vi "laser.vi"(8 "error in (no error)":errorcluster, 11 "this module name":string) -> (0 "error out":errorcluster)   [LabVIEW 2019]
doc: "Communicates with a laser to set the output power."
uses:
  common/common data types/common_event_data.ctl
panel:
  out "global stop?":bool
  in  "stop this module":bool
  out "targetted":bool
  out "msg target":string
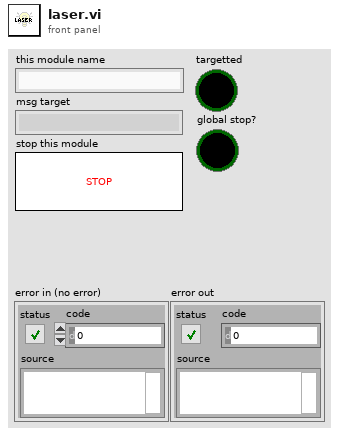
[diagram p1: front panel]
types:
  T1 = typedef "common_event_data.ctl" = cluster{"sender":string, "target":string, "msg":string, "data":variant}
  T2 = cluster{"this module name":string, "laser SP":dbl}
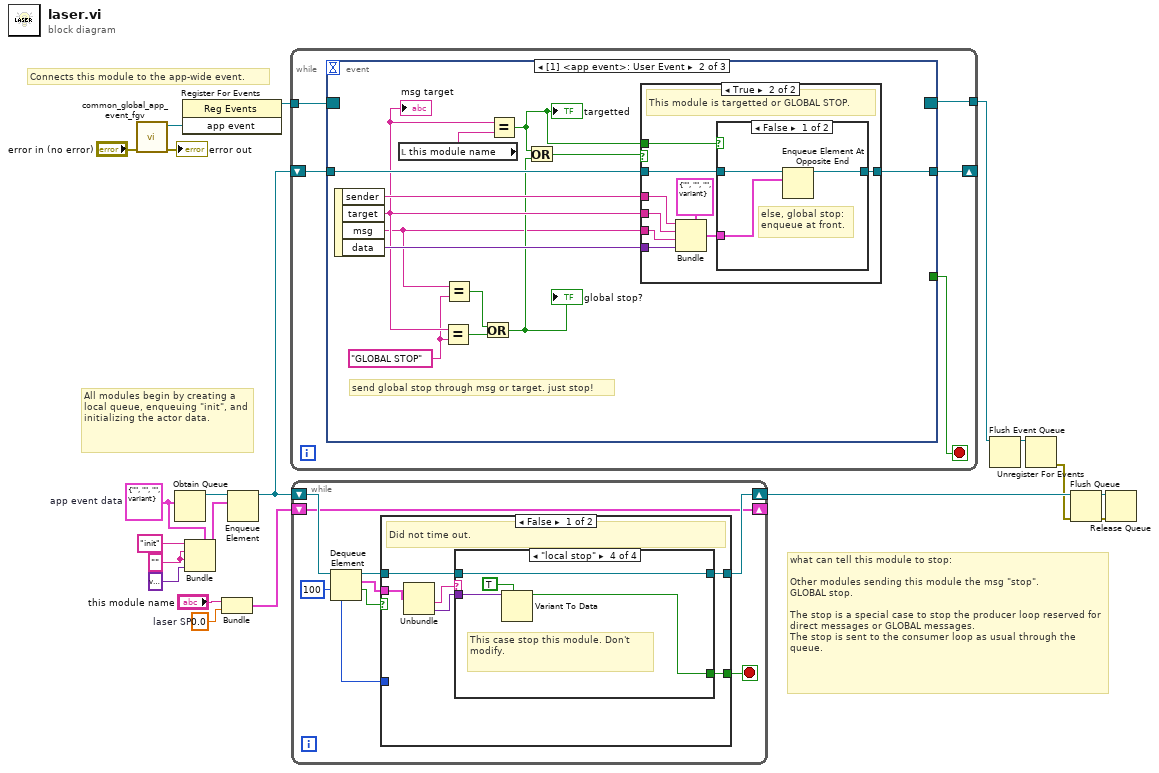
[diagram p0: block diagram]
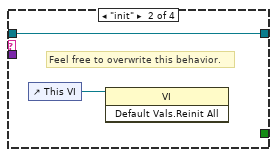
[diagram p3: hidden frame]
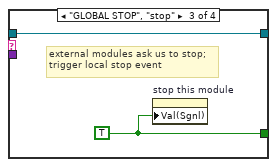
[diagram p4: hidden frame]
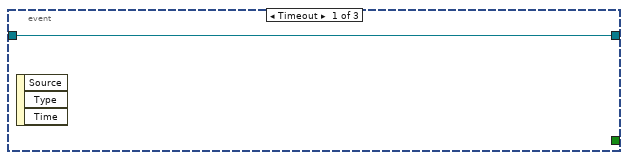
[diagram p6: hidden frame]
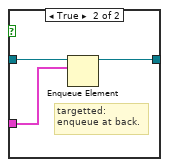
[diagram p8: hidden frame]
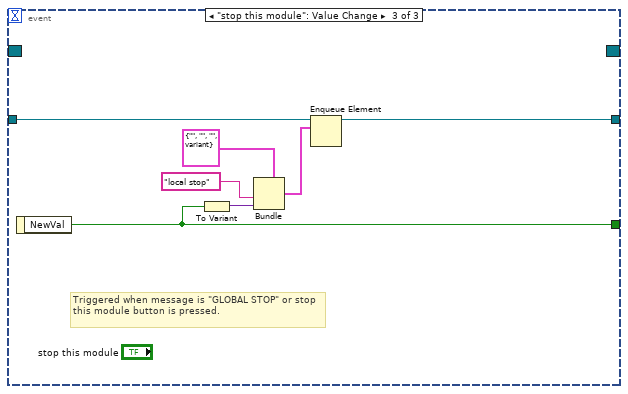
[diagram p9: hidden frame]
diagram:
  w1 = 0.0  # laser SP
  w6 = "" ("target")
  w8 = T1 {"sender"="", "target"="", "msg"="", "data"=variant}  # app event data
  # "All modules begin by creating a local queue, enqueuing \"init\", and initializing the actor data."
  # "what can tell this module to stop:\n\nOther modules sending this module the msg \"stop\".\nGLOBAL stop.\n\nThe stop is a special case to stop the producer loop reserved for direct messages or GLOBAL messages.\nThe stop is sent to the consumer loop as usual through the queue."
  # "Connects this module to the app-wide event."
  n1 = call "common_global_app_event_fgv.vi"("error in (no error)"="error in (no error)") -> ("error out"=→"error out":errorcluster, "app event"=w13:refnum<user-event>)  [unwired: 9 in]
  n2 = Obtain Queue(element data type=w8) -> (queue out=w20:refnum<queue>)  [unwired: 4 in, 2 out]
  n3 = register-events(w13) -> (reference out=w14:refnum<event-registration>)  [unwired: 2 in, 1 out]
  n4 = Bundle(cluster=w8, "sender"="init" ("msg"), "target"=w6, "msg"=w6, "data"=variant) -> (w18:T1)
  n5 = Bundle("this module name"="this module name", "laser SP"=w1) -> (w4:T2)  [unwired: 1 in]
  n6 = Enqueue Element(queue=w20, element=w18) -> (queue out=w17:refnum<queue>)  [unwired: 2 in, 2 out]
  n7 = while {
    tunnel: w14 -> [w25]
    shift-right: [w23] -> _
    shift-left: w17 -> [w24]
    tunnel: [w22] -> w3
    stop <- w21 stop-if-true
    n8 = event shown="[1] <app event>: User Event" {
      selector: w25 -> [_ _ _]
      dyn-events: [_ _ _] -> w22
      timeout: _ -> [_ _ _]
      tunnel: w24 -> [w26 w38 w60]
      tunnel: [w26 w37 w61] -> w23
      tunnel: [_ _ w56] -> w21
      event Timeout {
        n9 = event-data() -> ()  [unwired: 1 in, 3 out]
      }
      event User Event {
        w30 = "GLOBAL STOP"
        # "send global stop through msg or target. just stop!"
        n10 = event-data() -> ("sender"=w36:string, "target"=w35:string, "msg"=w29:string, "data"=w39:variant)  [unwired: 1 in]
        "msg target" <- w35
        n11 = local read "this module name"() -> (w27:string)
        n12 = Equal?(x=w35, y=w30) -> (x = y?=w32:bool)
        n13 = Equal?(x=w29, y=w30) -> (x = y?=w28:bool)
        n14 = Or(x=w28, y=w32) -> (x .or. y?=w31:bool)
        "global stop?" <- w31
        n15 = Equal?(x=w35, y=w27) -> (x = y?=w33:bool)
        "targetted" <- w33
        n16 = Or(x=w33, y=w31) -> (x .or. y?=w34:bool)
        n17 = case shown="True" w34 {
          tunnel: w29 -> [_ w45]
          tunnel: w39 -> [_ w46]
          tunnel: w38 -> [w40 w49]
          tunnel: [w40 w48] -> w37
          tunnel: w35 -> [_ w44]
          tunnel: w36 -> [_ w43]
          tunnel: w33 -> [_ w41]
          frame False {
          }
          frame True {
            # "This module is targetted or GLOBAL STOP."
            n18 = Bundle(cluster=T1 {"sender"="", "target"="", "msg"="", "data"=variant}, "sender"=w43, "target"=w44, "msg"=w45, "data"=w46) -> (w42:T1)
            n19 = case shown="False" w41 {
              tunnel: w49 -> [w52 w55]
              tunnel: [w51 w54] -> w48
              tunnel: w42 -> [w50 w53]
              frame False {
                # "else, global stop: \nenqueue at front."
                n20 = Enqueue Element At Opposite End(queue=w52, element=w50) -> (queue out=w51:refnum<queue>)  [unwired: 2 in, 2 out]
              }
              frame True {
                # "targetted:\nenqueue at back."
                n21 = Enqueue Element(queue=w55, element=w53) -> (queue out=w54:refnum<queue>)  [unwired: 2 in, 2 out]
              }
            }
          }
        }
      }
      event "stop this module": Value Change {
        # "Triggered when message is \"GLOBAL STOP\" or stop this module button is pressed."
        n22 = event-data() -> ("NewVal"=w56:bool)  [unwired: 1 in]
        n23 = To Variant(anything=w56) -> (Variant=w57:variant)
        n24 = Bundle(cluster=T1 {"sender"="", "target"="", "msg"="", "data"=variant}, "msg"="local stop", "data"=w57) -> (w62:T1)  [unwired: 2 in]
        n25 = Enqueue Element(queue=w60, element=w62) -> (queue out=w61:refnum<queue>)  [unwired: 2 in, 2 out]
      }
    }
  }
  n26 = while {
    shift-right: [w67] -> w15
    shift-left: w17 -> [w70]
    shift-right: [w64] -> _
    shift-left: w4 -> [w64]
    stop <- w66 stop-if-true
    w63 = 100 ("timeout in ms (-1)")
    n27 = Dequeue Element(queue=w70, timeout in ms (-1)=w63) -> (queue out=w68:refnum<queue>, element=w69:T1, timed out?=w65:bool)  [unwired: 1 in, 1 out]
    n28 = case shown="False" w65 {
      tunnel: w69 -> [w76 _]
      tunnel: w68 -> [w75 w86]
      tunnel: [w74 w86] -> w67
      tunnel: [w73 _] -> w66
      tunnel: w63 -> [_ _]
      frame False {
        # "Did not time out."
        n29 = Unbundle(w76) -> ("msg"=w71:string, "data"=w72:variant)  [unwired: 2 out]
        n30 = case shown="\"local stop\"" w71 {
          tunnel: w75 -> [w77 w79 w81 w85]
          tunnel: [w77 w79 w81 w85] -> w74
          tunnel: w72 -> [_ _ _ w83]
          tunnel: [_ _ w80 w82] -> w73
          frame Default {
            # "unsupported message."
          }
          frame "init" {
            # "Feel free to overwrite this behavior."
            n31 = control-ref of="This VI"() -> (w78:refnum<vi>)
            n32 = invoke class="VI" method="Default Vals.Reinit All"(reference=w78) -> ()  [unwired: 2 in, 3 out]
          }
          frame "GLOBAL STOP", "stop" {
            w80 = TRUE
            # "external modules ask us to stop;\ntrigger local stop event"
            n33 = property on="stop this module" class="Bool (strict)"("Val(Sgnl)"=w80) -> ()  [unwired: 2 in, 2 out]
          }
          frame "local stop" {
            # "This case stop this module. Don't modify."
            n34 = Variant To Data(type=TRUE, Variant=w83) -> (data=w82:bool)  [unwired: 1 in, 1 out]
          }
        }
      }
      frame True {
        # "Timed out. Do periodic stuff."
      }
    }
  }
  n35 = Flush Event Queue(0:w3) -> (8:w2:refnum<event-registration>)  [unwired: 5 in, 2 out]
  n36 = Unregister For Events(event registration refnum=w2) -> (error out=w10:errorcluster)  [unwired: 1 in]
  n37 = Flush Queue(queue=w15, error in (no error)=w10) -> (queue out=w16:refnum<queue>, error out=w9:errorcluster)  [unwired: 1 out]
  n38 = Release Queue(queue=w16, error in (no error)=w9) -> ()  [unwired: 1 in, 3 out]
